vi "Init Filters.vi"(6 "Fs":u32, 9 "PSD ref":refnum<vi>, 10 "BP Filter data":T2, 11 "Set":T1 {"PSD Filter"."Forward Coefficients" format="%.4f"; "PSD Filter"."Reverse Coefficients" format="%.4f"}) -> (3 "output cluster":T1 {"PSD Filter"."Forward Coefficients" format="%.4f"; "PSD Filter"."Reverse Coefficients" format="%.4f"})   [LabVIEW 2017, in "Processing.lvlib"]
uses:
  Processing.lvlib
  BP Filter Settings.ctl
  <vilib>/Analysis/3filter.llb/Filter Passband Type.ctl
  Filters.ctl
  <vilib>/Analysis/4window.llb/windowTd.ctl
  <vilib>/Analysis/4window.llb/Symmetric Window (DBL).vi
  <vilib>/Analysis/NI_AALPro.lvlib
  <vilib>/Analysis/NI_AALBase.lvlib
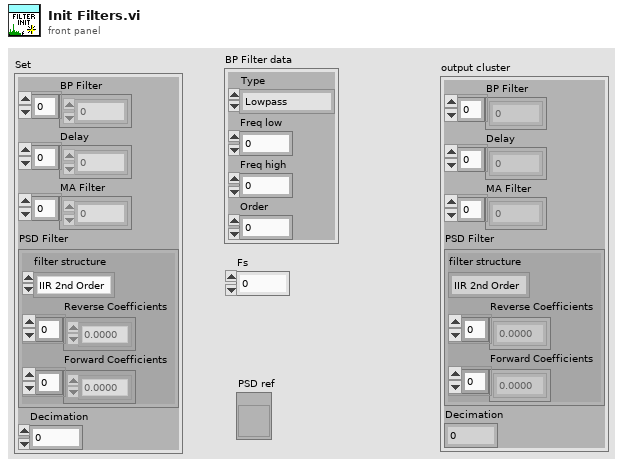
[diagram p1: front panel]
types:
  T1 = typedef "Processing.lvlib/Filters.ctl" = cluster{"BP Filter":dbl[], "Delay":dbl[], "MA Filter":dbl[], "PSD Filter":cluster{"filter structure":enum32{"IIR 2nd Order", "IIR 4th Order"}, "Reverse Coefficients":dbl[], "Forward Coefficients":dbl[]}, "Decimation":i32}
  T2 = typedef "Processing.lvlib/BP Filter Settings.ctl" = cluster{"Type":T3, "Freq low":dbl, "Freq high":dbl, "Order":i32}
  T3 = typedef "NI_AALBase.lvlib/Filter Passband Type.ctl" = enum32{"Lowpass", "Highpass", "Bandpass", "Bandstop"}
  T4 = typedef "NI_AALPro.lvlib/windowTd.ctl" = u32
  T5 = cluster{"filter structure":enum32{"IIR 2nd Order", "IIR 4th Order"}, "Reverse Coefficients":dbl[], "Forward Coefficients":dbl[]}
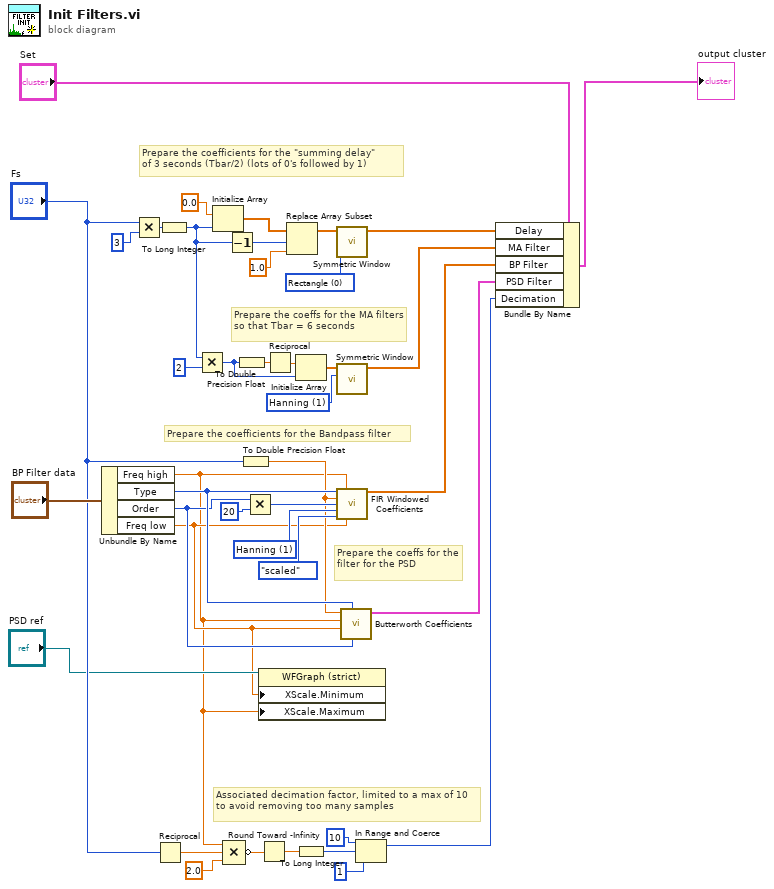
[diagram p0: block diagram]
diagram:
  w23 = T4 1 items=["Rectangle"=0, "Hanning"=1, "Hamming"=2, "Blackman-Harris"=3, "Exact Blackman"=4, "Blackman"=5, "Flat Top"=6, "4 Term B-Harris "=7, "7 Term B-Harris"=8, "Low Sidelobe"=9, "Blackman Nuttall"=11, "Triangle"=30, "Bartlett-Hanning"=31, "Bohman"=32, "Parzen"=33, "Welch"=34, "Kaiser"=60, "Dolph-Chebyshev"=61, "Gaussian"=62] ("window")
  w30 = T4 1 items=["Rectangle"=0, "Hanning"=1, "Hamming"=2, "Blackman-Harris"=3, "Exact Blackman"=4, "Blackman"=5, "Flat Top"=6, "4 Term B-Harris "=7, "7 Term B-Harris"=8, "Low Sidelobe"=9, "Blackman Nuttall"=11, "Triangle"=30, "Bartlett-Hanning"=31, "Bohman"=32, "Parzen"=33, "Welch"=34, "Kaiser"=60, "Dolph-Chebyshev"=61, "Gaussian"=62] ("window")
  w31 = T4 0 items=["Rectangle"=0, "Hanning"=1, "Hamming"=2, "Blackman-Harris"=3, "Exact Blackman"=4, "Blackman"=5, "Flat Top"=6, "4 Term B-Harris "=7, "7 Term B-Harris"=8, "Low Sidelobe"=9, "Blackman Nuttall"=11, "Triangle"=30, "Bartlett-Hanning"=31, "Bohman"=32, "Parzen"=33, "Welch"=34, "Kaiser"=60, "Dolph-Chebyshev"=61, "Gaussian"=62] ("window")
  # "Associated decimation factor, limited to a max of 10 to avoid removing too many samples"
  # "Prepare the coeffs for the filter for the PSD"
  # "Prepare the coefficients for the Bandpass filter"
  # "Prepare the coeffs for the MA filters so that Tbar = 6 seconds"
  # "Prepare the coefficients for the \"summing delay\" \nof 3 seconds (Tbar/2) (lots of 0's followed by 1)"
  n1 = Unbundle By Name("BP Filter data") -> ("Freq high"=w1:dbl, "Type"=w16:T3, "Order"=w15:i32, "Freq low"=w2:dbl)
  n2 = Multiply(x="Fs", y=u32 3 ("Numeric")) -> (x*y=w29:u32)
  n3 = Reciprocal(x="Fs") -> (1/x=w5:dbl)
  n4 = To Long Integer(number=w29) -> (32bit integer=w19:i32)
  n5 = Multiply(x=w19, y=2) -> (x*y=w27:i32)
  n6 = Initialize Array(0.0 ("element"), w19) -> (w40:dbl[])
  n7 = Compound Arithmetic op=MULTIPLY(w1, w5, 2.0 ("y")) -> (invert w8:dbl)
  n8 = Decrement(x=w19) -> (x-1=w18:i32)
  n9 = To Double Precision Float(number=w27) -> (double precision float=w32:dbl)
  n10 = To Double Precision Float(number="Fs") -> (double precision float=w14:dbl)
  n11 = Multiply(x=w15, y=20) -> (x*y=w22:i32)
  n12 = property on="Property Node" class="WFGraph (strict)"(reference="PSD ref", "XScale.Minimum"=w2, "XScale.Maximum"=w1) -> ()  [unwired: 1 in, 2 out]
  n13 = Round Toward -Infinity(1:w8) -> (0:w12:dbl)
  n14 = Reciprocal(x=w32) -> (1/x=w34:dbl)
  n15 = Replace Array Subset(array=w40, new element=1.0 ("new element/subarray"), index=w18) -> (w39:dbl[])
  n16 = Initialize Array(w34, w27) -> (w33:dbl[])
  n17 = To Long Integer(number=w12) -> (32bit integer=w10:i32)
  n18 = call-poly <vilib>:"Symmetric Window.vi"("window"=w31, "X"=w39) -> ("Windowed X"=w35:dbl[])  [unwired: 1 in, 8 out]
  n19 = call-poly <vilib>:"Symmetric Window.vi"("window"=w30, "X"=w33) -> ("Windowed X"=w26:dbl[])  [unwired: 1 in, 8 out]
  n20 = call <vilib>:"FIR Windowed Coefficients.vi"("filter type"=w16, "high cutoff freq: fh"=w1, "sampling freq: fs"=w14, "taps"=w22, "window"=w23, "option"=enum32{"not scaled", "scaled"}."scaled", "low cutoff freq: fl"=w2) -> ("FIR Windowed Coefficients"=w20:dbl[])  [unwired: 1 in, 7 out]
  n21 = call <vilib>:"Butterworth Coefficients.vi"("order"=w15, "filter type"=w16, "low cutoff freq: fl"=w2, "high cutoff freq: fh"=w1, "sampling freq: fs"=w14) -> ("IIR Filter Cluster"=w13:T5)  [unwired: 5 in, 1 out]
  n22 = In Range and Coerce(upper limit=10 ("y"), x=w10, lower limit=1 ("y")) -> (coerced(x)=w4:i32)  [unwired: 1 out]
  n23 = Bundle By Name(cluster="Set", "Delay"=w35, "MA Filter"=w26, "BP Filter"=w20, "PSD Filter"=w13, "Decimation"=w4) -> (→"output cluster":T1)
